vi "MenuConfiguration.vi"(7 "UserLevel":T1, 8 "ErrorIn":errorcluster, 11 "MenuRef":refnum<k9>) -> (0 "ErrorOut":errorcluster)   [LabVIEW 2018]
doc: "This VI configures the Run-Time menu(s) for the Main Panel depending on User Level. The Default settings has the Admin having access to the Configuration menu items while any other User Level (Operator) does not permit access to these menu items.\n\nCopyright © 2019 Epimedia, Inc. All Rights Reserved.\n\nThe Epimedia Application Library is Copyright © 2009-2017 Epimedia, Inc. \nAll Rights Reserved. Used under license."
uses:
  Controls/UserLevelEnum.ctl
panel:
  # "Copyright © 2019 Epimedia, Inc. All Rights Reserved.\n\nThe Epimedia Application Library is Copyright © 2009-2017 Epimedia, Inc. \nAll Rights Reserved. Used under license."
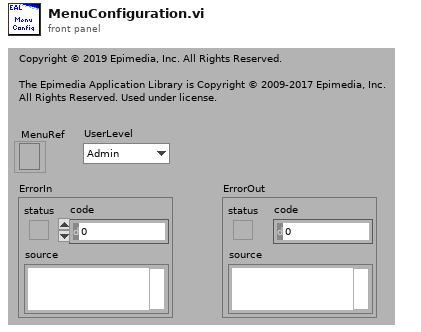
[diagram p1: front panel]
types:
  T1 = typedef "UserLevelEnum.ctl" = enum16{"Admin", "Operator"}
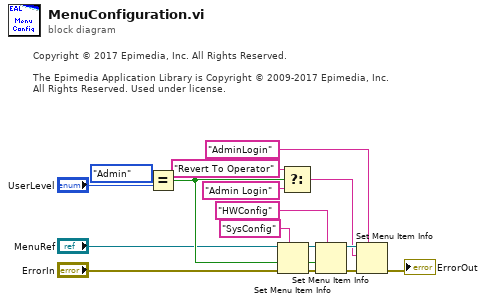
[diagram p0: block diagram]
diagram:
  # "Copyright © 2017 Epimedia, Inc. All Rights Reserved.\n\nThe Epimedia Application Library is Copyright © 2009-2017 Epimedia, Inc. \nAll Rights Reserved. Used under license."
  n1 = Equal?(x=UserLevelEnum."Admin", y="UserLevel") -> (x = y?=w4:bool)
  n2 = Set Menu Item Info(7:"SysConfig" ("item tag"), 8:"ErrorIn", 9:w4, 11:"MenuRef") -> (0:w11:errorcluster, 3:w15:refnum<k9>)  [unwired: 3 out]
  n3 = Select(t="Revert To Operator" ("item name"), s=w4, f="Admin Login" ("item name")) -> (s? t:f=w5:string)
  n4 = Set Menu Item Info(7:"HWConfig" ("item tag"), 8:w11, 9:w4, 11:w15) -> (0:w12:errorcluster, 3:w10:refnum<k9>)  [unwired: 3 out]
  n5 = Set Menu Item Info(7:"AdminLogin" ("item tag"), 8:w12, 10:w5, 11:w10) -> (0:→"ErrorOut":errorcluster)  [unwired: 4 out]
